vi "main(Test DQMH modules).bak.vi"() -> ()   [LabVIEW 2018, in "Application.lvlib"] (continued)
          tunnel: w8166 -> [w8203] mode=indexing
          tunnel: w8161 -> [w8204]
          tunnel: [w8200] -> w8164 mode=indexing
          n3766 = Unbundle By Name(w8203) -> ("command"=w8202:string, "command data"=w8201:variant)
          n3767 = call "App enquece.vi"("command data"=w8201, "command"=w8202, "queue in"=w8204) -> ("error out"=w8200:errorcluster)  [unwired: 7 in, 1 out]
        }
        n3768 = Merge Errors(w8165, w8164) -> (w8163:errorcluster)
      }
      frame "Test DRV 45A" {
        w8212 = T11 {"command"="", "command data"=variant} ("element")
        w8205 = 45 ("DUT index(0-59)")
        w8238 = T11 {"command"="", "command data"=variant} ("element")
        n3769 = disable-structure shown="LOGGING==TRUE" {
          disable-tunnel: w8216 -> [w8253 _]
          frame condition #0 (active) {
            n3770 = Empty String/Path?(string/path=w8253) -> (empty?=w8256:bool)
            n3771 = Select(t="Quece timeout", s=w8256, f=w8253) -> (s? t:f=w8252:string)
            n3772 = call "string log (SubVI).vi"("Enum"=enum16{"Init", "Log", "Read"}."Log", "state Name"=w8252) -> ()  [unwired: 8 in, 2 out]
          }
          frame condition #1 {
          }
        }
        n3773 = Flush Queue(queue=w8217) -> (queue out=w8218:refnum<queue>)  [unwired: 1 in, 2 out]
        n3774 = Decrement(x=w8205) -> (x-1=w8209:i32)
        n3775 = Index Array(array=w8206, index=w8209) -> (element=w8207:refnum<vi>)
        n3776 = property class="ColBox"(reference=w8207, "Value"=u32 10000536 ("DRV 1")) -> ()  [unwired: 1 in, 2 out]
        n3777 = To Variant(anything=bool[] [FALSE, FALSE, TRUE, FALSE, FALSE, FALSE]) -> (Variant=w8235:variant)
        n3778 = To Variant(anything=T6."demux1_10_channel8" ("demux1_10(x6)_encode")) -> (Variant=w8239:variant)
        n3779 = To Variant(anything=T4."mux6_1_channel3_3" ("mux6_1(3wires)_encode")) -> (Variant=w8242:variant)
        n3780 = To Variant(anything=T5."mux10_1_channel8" ("mux10_1(x6)_encode")) -> (Variant=w8244:variant)
        n3781 = Bundle By Name(cluster=w8238, "command"="MEAS.mux10-1", "command data"=w8244) -> (w8233:T11)
        n3782 = Bundle By Name(cluster=w8238, "command"="MEAS.mux6_1", "command data"=w8242) -> (w8232:T11)
        n3783 = Bundle By Name(cluster=w8238, "command"="MEAS.demux1-10", "command data"=w8239) -> (w8231:T11)
        n3784 = Bundle By Name(cluster=w8238, "command"="MEAS.eMIC", "command data"=w8235) -> (w8230:T11)
        n3785 = Bundle By Name(cluster=w8238, "command"="MEAS.AllRelaysOFF") -> (w8234:T11)
        n3786 = Build Array(w8234, w8233, w8232, w8231, w8230) -> (w8225:T11[])
        n3787 = Bundle By Name(cluster=w8212, "command"="MEAS.requestAC", "command data"=w8205) -> (w8226:T11)
        n3788 = Bundle By Name(cluster=w8212, "command"="Apps.WaitForEvent", "command data"=w8205) -> (w8211:T11)
        n3789 = Bundle By Name(cluster=w8212, "command"="MEAS.DMM dual read") -> (w8227:T11)
        n3790 = Bundle By Name(cluster=w8212, "command"="Apps.UI Update 1") -> (w8213:T11)
        n3791 = Build Array(w8227, w8226, w8211, w8213) -> (w8224:T11[])
        n3792 = Build Array (concatenate)(w8225, w8224) -> (w8223:T11[])
        n3793 = for {
          tunnel: w8223 -> [w8260] mode=indexing
          tunnel: w8218 -> [w8261]
          tunnel: [w8257] -> w8221 mode=indexing
          n3794 = Unbundle By Name(w8260) -> ("command"=w8259:string, "command data"=w8258:variant)
          n3795 = call "App enquece.vi"("command data"=w8258, "command"=w8259, "queue in"=w8261) -> ("error out"=w8257:errorcluster)  [unwired: 7 in, 1 out]
        }
        n3796 = Merge Errors(w8222, w8221) -> (w8220:errorcluster)
      }
      frame "Test DRV 46A" {
        w8269 = T11 {"command"="", "command data"=variant} ("element")
        w8263 = 46 ("DUT index(0-59)")
        w8295 = T11 {"command"="", "command data"=variant} ("element")
        n3797 = disable-structure shown="LOGGING==TRUE" {
          disable-tunnel: w8273 -> [w8310 _]
          frame condition #0 (active) {
            n3798 = Empty String/Path?(string/path=w8310) -> (empty?=w8313:bool)
            n3799 = Select(t="Quece timeout", s=w8313, f=w8310) -> (s? t:f=w8309:string)
            n3800 = call "string log (SubVI).vi"("Enum"=enum16{"Init", "Log", "Read"}."Log", "state Name"=w8309) -> ()  [unwired: 8 in, 2 out]
          }
          frame condition #1 {
          }
        }
        n3801 = Decrement(x=w8263) -> (x-1=w8266:i32)
        n3802 = Flush Queue(queue=w8274) -> (queue out=w8275:refnum<queue>)  [unwired: 1 in, 2 out]
        n3803 = Index Array(array=w8262, index=w8266) -> (element=w8264:refnum<vi>)
        n3804 = property class="ColBox"(reference=w8264, "Value"=u32 10000536 ("DRV 1")) -> ()  [unwired: 1 in, 2 out]
        n3805 = To Variant(anything=bool[] [FALSE, FALSE, TRUE, FALSE, FALSE, FALSE]) -> (Variant=w8292:variant)
        n3806 = To Variant(anything=T6."demux1_10_channel8" ("demux1_10(x6)_encode")) -> (Variant=w8296:variant)
        n3807 = To Variant(anything=T4."mux6_1_channel3_3" ("mux6_1(3wires)_encode")) -> (Variant=w8299:variant)
        n3808 = To Variant(anything=T5."mux10_1_channel8" ("mux10_1(x6)_encode")) -> (Variant=w8301:variant)
        n3809 = Bundle By Name(cluster=w8295, "command"="MEAS.mux10-1", "command data"=w8301) -> (w8290:T11)
        n3810 = Bundle By Name(cluster=w8295, "command"="MEAS.mux6_1", "command data"=w8299) -> (w8289:T11)
        n3811 = Bundle By Name(cluster=w8295, "command"="MEAS.demux1-10", "command data"=w8296) -> (w8288:T11)
        n3812 = Bundle By Name(cluster=w8295, "command"="MEAS.eMIC", "command data"=w8292) -> (w8287:T11)
        n3813 = Bundle By Name(cluster=w8295, "command"="MEAS.AllRelaysOFF") -> (w8291:T11)
        n3814 = Build Array(w8291, w8290, w8289, w8288, w8287) -> (w8282:T11[])
        n3815 = Bundle By Name(cluster=w8269, "command"="MEAS.requestAC", "command data"=w8263) -> (w8283:T11)
        n3816 = Bundle By Name(cluster=w8269, "command"="Apps.WaitForEvent", "command data"=w8263) -> (w8268:T11)
        n3817 = Bundle By Name(cluster=w8269, "command"="MEAS.DMM dual read") -> (w8284:T11)
        n3818 = Bundle By Name(cluster=w8269, "command"="Apps.UI Update 1") -> (w8270:T11)
        n3819 = Build Array(w8284, w8283, w8268, w8270) -> (w8281:T11[])
        n3820 = Build Array (concatenate)(w8282, w8281) -> (w8280:T11[])
        n3821 = for {
          tunnel: w8280 -> [w8317] mode=indexing
          tunnel: w8275 -> [w8318]
          tunnel: [w8314] -> w8278 mode=indexing
          n3822 = Unbundle By Name(w8317) -> ("command"=w8316:string, "command data"=w8315:variant)
          n3823 = call "App enquece.vi"("command data"=w8315, "command"=w8316, "queue in"=w8318) -> ("error out"=w8314:errorcluster)  [unwired: 7 in, 1 out]
        }
        n3824 = Merge Errors(w8279, w8278) -> (w8277:errorcluster)
      }
      frame "Test DRV 47A" {
        w8328 = T11 {"command"="", "command data"=variant} ("element")
        w8319 = 47 ("DUT index(0-59)")
        w8352 = T11 {"command"="", "command data"=variant} ("element")
        n3825 = disable-structure shown="LOGGING==TRUE" {
          disable-tunnel: w8332 -> [w8367 _]
          frame condition #0 (active) {
            n3826 = Empty String/Path?(string/path=w8367) -> (empty?=w8370:bool)
            n3827 = Select(t="Quece timeout", s=w8370, f=w8367) -> (s? t:f=w8366:string)
            n3828 = call "string log (SubVI).vi"("Enum"=enum16{"Init", "Log", "Read"}."Log", "state Name"=w8366) -> ()  [unwired: 8 in, 2 out]
          }
          frame condition #1 {
          }
        }
        n3829 = Decrement(x=w8319) -> (x-1=w8323:i32)
        n3830 = Flush Queue(queue=w8333) -> (queue out=w8334:refnum<queue>)  [unwired: 1 in, 2 out]
        n3831 = Index Array(array=w8320, index=w8323) -> (element=w8321:refnum<vi>)
        n3832 = property class="ColBox"(reference=w8321, "Value"=u32 10000536 ("DRV 1")) -> ()  [unwired: 1 in, 2 out]
        n3833 = To Variant(anything=bool[] [FALSE, FALSE, FALSE, FALSE, TRUE, FALSE]) -> (Variant=w8349:variant)
        n3834 = To Variant(anything=T6."demux1_10_channel8" ("demux1_10(x6)_encode")) -> (Variant=w8353:variant)
        n3835 = To Variant(anything=T4."mux6_1_channel5_3" ("mux6_1(3wires)_encode")) -> (Variant=w8356:variant)
        n3836 = To Variant(anything=T5."mux10_1_channel8" ("mux10_1(x6)_encode")) -> (Variant=w8358:variant)
        n3837 = Bundle By Name(cluster=w8352, "command"="MEAS.mux10-1", "command data"=w8358) -> (w8347:T11)
        n3838 = Bundle By Name(cluster=w8352, "command"="MEAS.mux6_1", "command data"=w8356) -> (w8346:T11)
        n3839 = Bundle By Name(cluster=w8352, "command"="MEAS.demux1-10", "command data"=w8353) -> (w8345:T11)
        n3840 = Bundle By Name(cluster=w8352, "command"="MEAS.eMIC", "command data"=w8349) -> (w8344:T11)
        n3841 = Bundle By Name(cluster=w8352, "command"="MEAS.AllRelaysOFF") -> (w8348:T11)
        n3842 = Build Array(w8348, w8347, w8346, w8345, w8344) -> (w8339:T11[])
        n3843 = Bundle By Name(cluster=w8328, "command"="MEAS.requestAC", "command data"=w8319) -> (w8340:T11)
        n3844 = Bundle By Name(cluster=w8328, "command"="Apps.WaitForEvent", "command data"=w8319) -> (w8327:T11)
        n3845 = Bundle By Name(cluster=w8328, "command"="Apps.UI Update 1") -> (w8329:T11)
        n3846 = Bundle By Name(cluster=w8328, "command"="MEAS.DMM dual read") -> (w8341:T11)
        n3847 = Build Array(w8341, w8340, w8327, w8329) -> (w8338:T11[])
        n3848 = Build Array (concatenate)(w8339, w8338) -> (w8337:T11[])
        n3849 = for {
          tunnel: w8337 -> [w8374] mode=indexing
          tunnel: w8334 -> [w8375]
          tunnel: [w8371] -> w8336 mode=indexing
          n3850 = Unbundle By Name(w8374) -> ("command"=w8373:string, "command data"=w8372:variant)
          n3851 = call "App enquece.vi"("command data"=w8372, "command"=w8373, "queue in"=w8375) -> ("error out"=w8371:errorcluster)  [unwired: 7 in, 1 out]
        }
        n3852 = Merge Errors(w8324, w8336) -> (w8335:errorcluster)
      }
      frame "Test DRV 48A" {
        w8383 = T11 {"command"="", "command data"=variant} ("element")
        w8377 = 48 ("DUT index(0-59)")
        w8409 = T11 {"command"="", "command data"=variant} ("element")
        n3853 = disable-structure shown="LOGGING==TRUE" {
          disable-tunnel: w8387 -> [w8424 _]
          frame condition #0 (active) {
            n3854 = Empty String/Path?(string/path=w8424) -> (empty?=w8427:bool)
            n3855 = Select(t="Quece timeout", s=w8427, f=w8424) -> (s? t:f=w8423:string)
            n3856 = call "string log (SubVI).vi"("Enum"=enum16{"Init", "Log", "Read"}."Log", "state Name"=w8423) -> ()  [unwired: 8 in, 2 out]
          }
          frame condition #1 {
          }
        }
        n3857 = Decrement(x=w8377) -> (x-1=w8380:i32)
        n3858 = Flush Queue(queue=w8388) -> (queue out=w8389:refnum<queue>)  [unwired: 1 in, 2 out]
        n3859 = Index Array(array=w8378, index=w8380) -> (element=w8376:refnum<vi>)
        n3860 = property class="ColBox"(reference=w8376, "Value"=u32 10000536 ("DRV 1")) -> ()  [unwired: 1 in, 2 out]
        n3861 = To Variant(anything=bool[] [FALSE, FALSE, FALSE, FALSE, FALSE, TRUE]) -> (Variant=w8406:variant)
        n3862 = To Variant(anything=T6."demux1_10_channel8" ("demux1_10(x6)_encode")) -> (Variant=w8410:variant)
        n3863 = To Variant(anything=T4."mux6_1_channel6_3" ("mux6_1(3wires)_encode")) -> (Variant=w8413:variant)
        n3864 = To Variant(anything=T5."mux10_1_channel8" ("mux10_1(x6)_encode")) -> (Variant=w8415:variant)
        n3865 = Bundle By Name(cluster=w8409, "command"="MEAS.mux10-1", "command data"=w8415) -> (w8404:T11)
        n3866 = Bundle By Name(cluster=w8409, "command"="MEAS.mux6_1", "command data"=w8413) -> (w8403:T11)
        n3867 = Bundle By Name(cluster=w8409, "command"="MEAS.demux1-10", "command data"=w8410) -> (w8402:T11)
        n3868 = Bundle By Name(cluster=w8409, "command"="MEAS.eMIC", "command data"=w8406) -> (w8401:T11)
        n3869 = Bundle By Name(cluster=w8409, "command"="MEAS.AllRelaysOFF") -> (w8405:T11)
        n3870 = Build Array(w8405, w8404, w8403, w8402, w8401) -> (w8396:T11[])
        n3871 = Bundle By Name(cluster=w8383, "command"="MEAS.requestAC", "command data"=w8377) -> (w8397:T11)
        n3872 = Bundle By Name(cluster=w8383, "command"="Apps.WaitForEvent", "command data"=w8377) -> (w8382:T11)
        n3873 = Bundle By Name(cluster=w8383, "command"="MEAS.DMM dual read") -> (w8398:T11)
        n3874 = Bundle By Name(cluster=w8383, "command"="Apps.UI Update 1") -> (w8384:T11)
        n3875 = Build Array(w8398, w8397, w8382, w8384) -> (w8395:T11[])
        n3876 = Build Array (concatenate)(w8396, w8395) -> (w8394:T11[])
        n3877 = for {
          tunnel: w8394 -> [w8431] mode=indexing
          tunnel: w8389 -> [w8432]
          tunnel: [w8428] -> w8392 mode=indexing
          n3878 = Unbundle By Name(w8431) -> ("command"=w8430:string, "command data"=w8429:variant)
          n3879 = call "App enquece.vi"("command data"=w8429, "command"=w8430, "queue in"=w8432) -> ("error out"=w8428:errorcluster)  [unwired: 7 in, 1 out]
        }
        n3880 = Merge Errors(w8393, w8392) -> (w8391:errorcluster)
      }
      frame "Test DRV 49A" {
        w8440 = T11 {"command"="", "command data"=variant} ("element")
        w8434 = 49 ("DUT index(0-59)")
        w8466 = T11 {"command"="", "command data"=variant} ("element")
        n3881 = disable-structure shown="LOGGING==TRUE" {
          disable-tunnel: w8444 -> [w8481 _]
          frame condition #0 (active) {
            n3882 = Empty String/Path?(string/path=w8481) -> (empty?=w8484:bool)
            n3883 = Select(t="Quece timeout", s=w8484, f=w8481) -> (s? t:f=w8480:string)
            n3884 = call "string log (SubVI).vi"("Enum"=enum16{"Init", "Log", "Read"}."Log", "state Name"=w8480) -> ()  [unwired: 8 in, 2 out]
          }
          frame condition #1 {
          }
        }
        n3885 = Flush Queue(queue=w8445) -> (queue out=w8446:refnum<queue>)  [unwired: 1 in, 2 out]
        n3886 = Decrement(x=w8434) -> (x-1=w8437:i32)
        n3887 = Index Array(array=w8435, index=w8437) -> (element=w8433:refnum<vi>)
        n3888 = property class="ColBox"(reference=w8433, "Value"=u32 10000536 ("DRV 1")) -> ()  [unwired: 1 in, 2 out]
        n3889 = To Variant(anything=bool[] [TRUE, FALSE, FALSE, FALSE, FALSE, FALSE]) -> (Variant=w8463:variant)
        n3890 = To Variant(anything=T6."demux1_10_channel9" ("demux1_10(x6)_encode")) -> (Variant=w8467:variant)
        n3891 = To Variant(anything=T4."mux6_1_channel1_3" ("mux6_1(3wires)_encode")) -> (Variant=w8470:variant)
        n3892 = To Variant(anything=T5."mux10_1_channel9" ("mux10_1(x6)_encode")) -> (Variant=w8472:variant)
        n3893 = Bundle By Name(cluster=w8466, "command"="MEAS.mux10-1", "command data"=w8472) -> (w8461:T11)
        n3894 = Bundle By Name(cluster=w8466, "command"="MEAS.mux6_1", "command data"=w8470) -> (w8460:T11)
        n3895 = Bundle By Name(cluster=w8466, "command"="MEAS.demux1-10", "command data"=w8467) -> (w8459:T11)
        n3896 = Bundle By Name(cluster=w8466, "command"="MEAS.eMIC", "command data"=w8463) -> (w8458:T11)
        n3897 = Bundle By Name(cluster=w8466, "command"="MEAS.AllRelaysOFF") -> (w8462:T11)
        n3898 = Build Array(w8462, w8461, w8460, w8459, w8458) -> (w8453:T11[])
        n3899 = Bundle By Name(cluster=w8440, "command"="MEAS.requestAC", "command data"=w8434) -> (w8454:T11)
        n3900 = Bundle By Name(cluster=w8440, "command"="Apps.WaitForEvent", "command data"=w8434) -> (w8439:T11)
        n3901 = Bundle By Name(cluster=w8440, "command"="MEAS.DMM dual read") -> (w8455:T11)
        n3902 = Bundle By Name(cluster=w8440, "command"="Apps.UI Update 1") -> (w8441:T11)
        n3903 = Build Array(w8455, w8454, w8439, w8441) -> (w8452:T11[])
        n3904 = Build Array (concatenate)(w8453, w8452) -> (w8451:T11[])
        n3905 = for {
          tunnel: w8451 -> [w8488] mode=indexing
          tunnel: w8446 -> [w8489]
          tunnel: [w8485] -> w8449 mode=indexing
          n3906 = Unbundle By Name(w8488) -> ("command"=w8487:string, "command data"=w8486:variant)
          n3907 = call "App enquece.vi"("command data"=w8486, "command"=w8487, "queue in"=w8489) -> ("error out"=w8485:errorcluster)  [unwired: 7 in, 1 out]
        }
        n3908 = Merge Errors(w8450, w8449) -> (w8448:errorcluster)
      }
      frame "Test DRV 50A" {
        w8497 = T11 {"command"="", "command data"=variant} ("element")
        w8491 = 50 ("DUT index(0-59)")
        w8523 = T11 {"command"="", "command data"=variant} ("element")
        n3909 = disable-structure shown="LOGGING==TRUE" {
          disable-tunnel: w8501 -> [w8538 _]
          frame condition #0 (active) {
            n3910 = Empty String/Path?(string/path=w8538) -> (empty?=w8541:bool)
            n3911 = Select(t="Quece timeout", s=w8541, f=w8538) -> (s? t:f=w8537:string)
            n3912 = call "string log (SubVI).vi"("Enum"=enum16{"Init", "Log", "Read"}."Log", "state Name"=w8537) -> ()  [unwired: 8 in, 2 out]
          }
          frame condition #1 {
          }
        }
        n3913 = Flush Queue(queue=w8502) -> (queue out=w8503:refnum<queue>)  [unwired: 1 in, 2 out]
        n3914 = Decrement(x=w8491) -> (x-1=w8494:i32)
        n3915 = Index Array(array=w8492, index=w8494) -> (element=w8490:refnum<vi>)
        n3916 = property class="ColBox"(reference=w8490, "Value"=u32 10000536 ("DRV 1")) -> ()  [unwired: 1 in, 2 out]
        n3917 = To Variant(anything=bool[] [FALSE, TRUE, FALSE, FALSE, FALSE, FALSE]) -> (Variant=w8520:variant)
        n3918 = To Variant(anything=T6."demux1_10_channel9" ("demux1_10(x6)_encode")) -> (Variant=w8524:variant)
        n3919 = To Variant(anything=T4."mux6_1_channel2_3" ("mux6_1(3wires)_encode")) -> (Variant=w8527:variant)
        n3920 = To Variant(anything=T5."mux10_1_channel9" ("mux10_1(x6)_encode")) -> (Variant=w8529:variant)
        n3921 = Bundle By Name(cluster=w8523, "command"="MEAS.mux10-1", "command data"=w8529) -> (w8518:T11)
        n3922 = Bundle By Name(cluster=w8523, "command"="MEAS.mux6_1", "command data"=w8527) -> (w8517:T11)
        n3923 = Bundle By Name(cluster=w8523, "command"="MEAS.demux1-10", "command data"=w8524) -> (w8516:T11)
        n3924 = Bundle By Name(cluster=w8523, "command"="MEAS.eMIC", "command data"=w8520) -> (w8515:T11)
        n3925 = Bundle By Name(cluster=w8523, "command"="MEAS.AllRelaysOFF") -> (w8519:T11)
        n3926 = Build Array(w8519, w8518, w8517, w8516, w8515) -> (w8510:T11[])
        n3927 = Bundle By Name(cluster=w8497, "command"="MEAS.requestAC", "command data"=w8491) -> (w8511:T11)
        n3928 = Bundle By Name(cluster=w8497, "command"="Apps.WaitForEvent", "command data"=w8491) -> (w8496:T11)
        n3929 = Bundle By Name(cluster=w8497, "command"="MEAS.DMM dual read") -> (w8512:T11)
        n3930 = Bundle By Name(cluster=w8497, "command"="Apps.UI Update 1") -> (w8498:T11)
        n3931 = Build Array(w8512, w8511, w8496, w8498) -> (w8509:T11[])
        n3932 = Build Array (concatenate)(w8510, w8509) -> (w8508:T11[])
        n3933 = for {
          tunnel: w8508 -> [w8545] mode=indexing
          tunnel: w8503 -> [w8546]
          tunnel: [w8542] -> w8506 mode=indexing
          n3934 = Unbundle By Name(w8545) -> ("command"=w8544:string, "command data"=w8543:variant)
          n3935 = call "App enquece.vi"("command data"=w8543, "command"=w8544, "queue in"=w8546) -> ("error out"=w8542:errorcluster)  [unwired: 7 in, 1 out]
        }
        n3936 = Merge Errors(w8507, w8506) -> (w8505:errorcluster)
      }
      frame "Test DRV 51A" {
        w8554 = T11 {"command"="", "command data"=variant} ("element")
        w8547 = 51 ("DUT index(0-59)")
        w8580 = T11 {"command"="", "command data"=variant} ("element")
        n3937 = disable-structure shown="LOGGING==TRUE" {
          disable-tunnel: w8558 -> [w8595 _]
          frame condition #0 (active) {
            n3938 = Empty String/Path?(string/path=w8595) -> (empty?=w8598:bool)
            n3939 = Select(t="Quece timeout", s=w8598, f=w8595) -> (s? t:f=w8594:string)
            n3940 = call "string log (SubVI).vi"("Enum"=enum16{"Init", "Log", "Read"}."Log", "state Name"=w8594) -> ()  [unwired: 8 in, 2 out]
          }
          frame condition #1 {
          }
        }
        n3941 = Flush Queue(queue=w8559) -> (queue out=w8560:refnum<queue>)  [unwired: 1 in, 2 out]
        n3942 = Decrement(x=w8547) -> (x-1=w8551:i32)
        n3943 = Index Array(array=w8548, index=w8551) -> (element=w8549:refnum<vi>)
        n3944 = property class="ColBox"(reference=w8549, "Value"=u32 10000536 ("DRV 1")) -> ()  [unwired: 1 in, 2 out]
        n3945 = To Variant(anything=bool[] [FALSE, FALSE, TRUE, FALSE, FALSE, FALSE]) -> (Variant=w8577:variant)
        n3946 = To Variant(anything=T6."demux1_10_channel9" ("demux1_10(x6)_encode")) -> (Variant=w8581:variant)
        n3947 = To Variant(anything=T4."mux6_1_channel3_3" ("mux6_1(3wires)_encode")) -> (Variant=w8584:variant)
        n3948 = To Variant(anything=T5."mux10_1_channel9" ("mux10_1(x6)_encode")) -> (Variant=w8586:variant)
        n3949 = Bundle By Name(cluster=w8580, "command"="MEAS.mux10-1", "command data"=w8586) -> (w8575:T11)
        n3950 = Bundle By Name(cluster=w8580, "command"="MEAS.mux6_1", "command data"=w8584) -> (w8574:T11)
        n3951 = Bundle By Name(cluster=w8580, "command"="MEAS.demux1-10", "command data"=w8581) -> (w8573:T11)
        n3952 = Bundle By Name(cluster=w8580, "command"="MEAS.eMIC", "command data"=w8577) -> (w8572:T11)
        n3953 = Bundle By Name(cluster=w8580, "command"="MEAS.AllRelaysOFF") -> (w8576:T11)
        n3954 = Build Array(w8576, w8575, w8574, w8573, w8572) -> (w8567:T11[])
        n3955 = Bundle By Name(cluster=w8554, "command"="MEAS.requestAC", "command data"=w8547) -> (w8568:T11)
        n3956 = Bundle By Name(cluster=w8554, "command"="Apps.WaitForEvent", "command data"=w8547) -> (w8553:T11)
        n3957 = Bundle By Name(cluster=w8554, "command"="MEAS.DMM dual read") -> (w8569:T11)
        n3958 = Bundle By Name(cluster=w8554, "command"="Apps.UI Update 1") -> (w8555:T11)
        n3959 = Build Array(w8569, w8568, w8553, w8555) -> (w8566:T11[])
        n3960 = Build Array (concatenate)(w8567, w8566) -> (w8565:T11[])
        n3961 = for {
          tunnel: w8565 -> [w8602] mode=indexing
          tunnel: w8560 -> [w8603]
          tunnel: [w8599] -> w8563 mode=indexing
          n3962 = Unbundle By Name(w8602) -> ("command"=w8601:string, "command data"=w8600:variant)
          n3963 = call "App enquece.vi"("command data"=w8600, "command"=w8601, "queue in"=w8603) -> ("error out"=w8599:errorcluster)  [unwired: 7 in, 1 out]
        }
        n3964 = Merge Errors(w8564, w8563) -> (w8562:errorcluster)
      }
      frame "Test DRV 52A" {
        w8611 = T11 {"command"="", "command data"=variant} ("element")
        w8604 = 52 ("DUT index(0-59)")
        w8637 = T11 {"command"="", "command data"=variant} ("element")
        n3965 = disable-structure shown="LOGGING==TRUE" {
          disable-tunnel: w8615 -> [w8652 _]
          frame condition #0 (active) {
            n3966 = Empty String/Path?(string/path=w8652) -> (empty?=w8655:bool)
            n3967 = Select(t="Quece timeout", s=w8655, f=w8652) -> (s? t:f=w8651:string)
            n3968 = call "string log (SubVI).vi"("Enum"=enum16{"Init", "Log", "Read"}."Log", "state Name"=w8651) -> ()  [unwired: 8 in, 2 out]
          }
          frame condition #1 {
          }
        }
        n3969 = Flush Queue(queue=w8616) -> (queue out=w8617:refnum<queue>)  [unwired: 1 in, 2 out]
        n3970 = Decrement(x=w8604) -> (x-1=w8608:i32)
        n3971 = Index Array(array=w8605, index=w8608) -> (element=w8606:refnum<vi>)
        n3972 = property class="ColBox"(reference=w8606, "Value"=u32 10000536 ("DRV 1")) -> ()  [unwired: 1 in, 2 out]
        n3973 = To Variant(anything=bool[] [FALSE, FALSE, FALSE, TRUE, FALSE, FALSE]) -> (Variant=w8634:variant)
        n3974 = To Variant(anything=T6."demux1_10_channel9" ("demux1_10(x6)_encode")) -> (Variant=w8638:variant)
        n3975 = To Variant(anything=T4."mux6_1_channel4_3" ("mux6_1(3wires)_encode")) -> (Variant=w8641:variant)
        n3976 = To Variant(anything=T5."mux10_1_channel9" ("mux10_1(x6)_encode")) -> (Variant=w8643:variant)
        n3977 = Bundle By Name(cluster=w8637, "command"="MEAS.mux10-1", "command data"=w8643) -> (w8632:T11)
        n3978 = Bundle By Name(cluster=w8637, "command"="MEAS.mux6_1", "command data"=w8641) -> (w8631:T11)
        n3979 = Bundle By Name(cluster=w8637, "command"="MEAS.demux1-10", "command data"=w8638) -> (w8630:T11)
        n3980 = Bundle By Name(cluster=w8637, "command"="MEAS.eMIC", "command data"=w8634) -> (w8629:T11)
        n3981 = Bundle By Name(cluster=w8637, "command"="MEAS.AllRelaysOFF") -> (w8633:T11)
        n3982 = Build Array(w8633, w8632, w8631, w8630, w8629) -> (w8624:T11[])
        n3983 = Bundle By Name(cluster=w8611, "command"="MEAS.requestAC", "command data"=w8604) -> (w8625:T11)
        n3984 = Bundle By Name(cluster=w8611, "command"="Apps.WaitForEvent", "command data"=w8604) -> (w8610:T11)
        n3985 = Bundle By Name(cluster=w8611, "command"="MEAS.DMM dual read") -> (w8626:T11)
        n3986 = Bundle By Name(cluster=w8611, "command"="Apps.UI Update 1") -> (w8612:T11)
        n3987 = Build Array(w8626, w8625, w8610, w8612) -> (w8623:T11[])
        n3988 = Build Array (concatenate)(w8624, w8623) -> (w8622:T11[])
        n3989 = for {
          tunnel: w8622 -> [w8659] mode=indexing
          tunnel: w8617 -> [w8660]
          tunnel: [w8656] -> w8620 mode=indexing
          n3990 = Unbundle By Name(w8659) -> ("command"=w8658:string, "command data"=w8657:variant)
          n3991 = call "App enquece.vi"("command data"=w8657, "command"=w8658, "queue in"=w8660) -> ("error out"=w8656:errorcluster)  [unwired: 7 in, 1 out]
        }
        n3992 = Merge Errors(w8621, w8620) -> (w8619:errorcluster)
      }
      frame "Test DRV 53A" {
        w8669 = T11 {"command"="", "command data"=variant} ("element")
        w8661 = 53 ("DUT index(0-59)")
        w8694 = T11 {"command"="", "command data"=variant} ("element")
        n3993 = disable-structure shown="LOGGING==TRUE" {
          disable-tunnel: w8673 -> [w8709 _]
          frame condition #0 (active) {
            n3994 = Empty String/Path?(string/path=w8709) -> (empty?=w8712:bool)
            n3995 = Select(t="Quece timeout", s=w8712, f=w8709) -> (s? t:f=w8708:string)
            n3996 = call "string log (SubVI).vi"("Enum"=enum16{"Init", "Log", "Read"}."Log", "state Name"=w8708) -> ()  [unwired: 8 in, 2 out]
          }
          frame condition #1 {
          }
        }
        n3997 = Flush Queue(queue=w8674) -> (queue out=w8675:refnum<queue>)  [unwired: 1 in, 2 out]
        n3998 = Decrement(x=w8661) -> (x-1=w8665:i32)
        n3999 = Index Array(array=w8662, index=w8665) -> (element=w8663:refnum<vi>)
        n4000 = property class="ColBox"(reference=w8663, "Value"=u32 10000536 ("DRV 1")) -> ()  [unwired: 1 in, 2 out]
        n4001 = To Variant(anything=bool[] [FALSE, FALSE, FALSE, FALSE, TRUE, FALSE]) -> (Variant=w8691:variant)
        n4002 = To Variant(anything=T6."demux1_10_channel9" ("demux1_10(x6)_encode")) -> (Variant=w8695:variant)
        n4003 = To Variant(anything=T4."mux6_1_channel5_3" ("mux6_1(3wires)_encode")) -> (Variant=w8698:variant)
        n4004 = To Variant(anything=T5."mux10_1_channel9" ("mux10_1(x6)_encode")) -> (Variant=w8700:variant)
        n4005 = Bundle By Name(cluster=w8694, "command"="MEAS.mux10-1", "command data"=w8700) -> (w8689:T11)
        n4006 = Bundle By Name(cluster=w8694, "command"="MEAS.mux6_1", "command data"=w8698) -> (w8688:T11)
        n4007 = Bundle By Name(cluster=w8694, "command"="MEAS.demux1-10", "command data"=w8695) -> (w8687:T11)
        n4008 = Bundle By Name(cluster=w8694, "command"="MEAS.eMIC", "command data"=w8691) -> (w8686:T11)
        n4009 = Bundle By Name(cluster=w8694, "command"="MEAS.AllRelaysOFF") -> (w8690:T11)
        n4010 = Build Array(w8690, w8689, w8688, w8687, w8686) -> (w8682:T11[])
        n4011 = Bundle By Name(cluster=w8669, "command"="MEAS.requestAC", "command data"=w8661) -> (w8683:T11)
        n4012 = Bundle By Name(cluster=w8669, "command"="Apps.WaitForEvent", "command data"=w8661) -> (w8668:T11)
        n4013 = Bundle By Name(cluster=w8669, "command"="MEAS.DMM dual read") -> (w8684:T11)
        n4014 = Bundle By Name(cluster=w8669, "command"="Apps.UI Update 1") -> (w8670:T11)
        n4015 = Build Array(w8684, w8683, w8668, w8670) -> (w8681:T11[])
        n4016 = Build Array (concatenate)(w8682, w8681) -> (w8680:T11[])
        n4017 = for {
          tunnel: w8680 -> [w8716] mode=indexing
          tunnel: w8675 -> [w8717]
          tunnel: [w8713] -> w8678 mode=indexing
          n4018 = Unbundle By Name(w8716) -> ("command"=w8715:string, "command data"=w8714:variant)
          n4019 = call "App enquece.vi"("command data"=w8714, "command"=w8715, "queue in"=w8717) -> ("error out"=w8713:errorcluster)  [unwired: 7 in, 1 out]
        }
        n4020 = Merge Errors(w8679, w8678) -> (w8677:errorcluster)
      }
      frame "Test DRV 54A" {
        w8725 = T11 {"command"="", "command data"=variant} ("element")
        w8718 = 54 ("DUT index(0-59)")
        w8751 = T11 {"command"="", "command data"=variant} ("element")
        n4021 = disable-structure shown="LOGGING==TRUE" {
          disable-tunnel: w8729 -> [w8766 _]
          frame condition #0 (active) {
            n4022 = Empty String/Path?(string/path=w8766) -> (empty?=w8769:bool)
            n4023 = Select(t="Quece timeout", s=w8769, f=w8766) -> (s? t:f=w8765:string)
            n4024 = call "string log (SubVI).vi"("Enum"=enum16{"Init", "Log", "Read"}."Log", "state Name"=w8765) -> ()  [unwired: 8 in, 2 out]
          }
          frame condition #1 {
          }
        }
        n4025 = Flush Queue(queue=w8730) -> (queue out=w8731:refnum<queue>)  [unwired: 1 in, 2 out]
        n4026 = Decrement(x=w8718) -> (x-1=w8722:i32)
        n4027 = Index Array(array=w8719, index=w8722) -> (element=w8720:refnum<vi>)
        n4028 = property class="ColBox"(reference=w8720, "Value"=u32 10000536 ("DRV 1")) -> ()  [unwired: 1 in, 2 out]
        n4029 = To Variant(anything=bool[] [FALSE, FALSE, FALSE, FALSE, FALSE, TRUE]) -> (Variant=w8748:variant)
        n4030 = To Variant(anything=T6."demux1_10_channel9" ("demux1_10(x6)_encode")) -> (Variant=w8752:variant)
        n4031 = To Variant(anything=T4."mux6_1_channel6_3" ("mux6_1(3wires)_encode")) -> (Variant=w8755:variant)
        n4032 = To Variant(anything=T5."mux10_1_channel9" ("mux10_1(x6)_encode")) -> (Variant=w8757:variant)
        n4033 = Bundle By Name(cluster=w8751, "command"="MEAS.mux10-1", "command data"=w8757) -> (w8746:T11)
        n4034 = Bundle By Name(cluster=w8751, "command"="MEAS.mux6_1", "command data"=w8755) -> (w8745:T11)
        n4035 = Bundle By Name(cluster=w8751, "command"="MEAS.demux1-10", "command data"=w8752) -> (w8744:T11)
        n4036 = Bundle By Name(cluster=w8751, "command"="MEAS.eMIC", "command data"=w8748) -> (w8743:T11)
        n4037 = Bundle By Name(cluster=w8751, "command"="MEAS.AllRelaysOFF") -> (w8747:T11)
        n4038 = Build Array(w8747, w8746, w8745, w8744, w8743) -> (w8738:T11[])
        n4039 = Bundle By Name(cluster=w8725, "command"="MEAS.requestAC", "command data"=w8718) -> (w8739:T11)
        n4040 = Bundle By Name(cluster=w8725, "command"="Apps.WaitForEvent", "command data"=w8718) -> (w8724:T11)
        n4041 = Bundle By Name(cluster=w8725, "command"="MEAS.DMM dual read") -> (w8740:T11)
        n4042 = Bundle By Name(cluster=w8725, "command"="Apps.UI Update 1") -> (w8726:T11)
        n4043 = Build Array(w8740, w8739, w8724, w8726) -> (w8737:T11[])
        n4044 = Build Array (concatenate)(w8738, w8737) -> (w8736:T11[])
        n4045 = for {
          tunnel: w8736 -> [w8773] mode=indexing
          tunnel: w8731 -> [w8774]
          tunnel: [w8770] -> w8734 mode=indexing
          n4046 = Unbundle By Name(w8773) -> ("command"=w8772:string, "command data"=w8771:variant)
          n4047 = call "App enquece.vi"("command data"=w8771, "command"=w8772, "queue in"=w8774) -> ("error out"=w8770:errorcluster)  [unwired: 7 in, 1 out]
        }
        n4048 = Merge Errors(w8735, w8734) -> (w8733:errorcluster)
      }
      frame "Test DRV 55A" {
        w8782 = T11 {"command"="", "command data"=variant} ("element")
        w8775 = 55 ("DUT index(0-59)")
        w8808 = T11 {"command"="", "command data"=variant} ("element")
        n4049 = disable-structure shown="LOGGING==TRUE" {
          disable-tunnel: w8786 -> [w8823 _]
          frame condition #0 (active) {
            n4050 = Empty String/Path?(string/path=w8823) -> (empty?=w8826:bool)
            n4051 = Select(t="Quece timeout", s=w8826, f=w8823) -> (s? t:f=w8822:string)
            n4052 = call "string log (SubVI).vi"("Enum"=enum16{"Init", "Log", "Read"}."Log", "state Name"=w8822) -> ()  [unwired: 8 in, 2 out]
          }
          frame condition #1 {
          }
        }
        n4053 = Flush Queue(queue=w8787) -> (queue out=w8788:refnum<queue>)  [unwired: 1 in, 2 out]
        n4054 = Decrement(x=w8775) -> (x-1=w8779:i32)
        n4055 = Index Array(array=w8776, index=w8779) -> (element=w8777:refnum<vi>)
        n4056 = property class="ColBox"(reference=w8777, "Value"=u32 10000536 ("DRV 1")) -> ()  [unwired: 1 in, 2 out]
        n4057 = To Variant(anything=bool[] [TRUE, FALSE, FALSE, FALSE, FALSE, FALSE]) -> (Variant=w8805:variant)
        n4058 = To Variant(anything=T6."demux1_10_channel10" ("demux1_10(x6)_encode")) -> (Variant=w8809:variant)
        n4059 = To Variant(anything=T4."mux6_1_channel1_3" ("mux6_1(3wires)_encode")) -> (Variant=w8812:variant)
        n4060 = To Variant(anything=T5."mux10_1_channel10" ("mux10_1(x6)_encode")) -> (Variant=w8814:variant)
        n4061 = Bundle By Name(cluster=w8808, "command"="MEAS.mux10-1", "command data"=w8814) -> (w8803:T11)
        n4062 = Bundle By Name(cluster=w8808, "command"="MEAS.mux6_1", "command data"=w8812) -> (w8802:T11)
        n4063 = Bundle By Name(cluster=w8808, "command"="MEAS.demux1-10", "command data"=w8809) -> (w8801:T11)
        n4064 = Bundle By Name(cluster=w8808, "command"="MEAS.eMIC", "command data"=w8805) -> (w8800:T11)
        n4065 = Bundle By Name(cluster=w8808, "command"="MEAS.AllRelaysOFF") -> (w8804:T11)
        n4066 = Build Array(w8804, w8803, w8802, w8801, w8800) -> (w8795:T11[])
        n4067 = Bundle By Name(cluster=w8782, "command"="MEAS.requestAC", "command data"=w8775) -> (w8796:T11)
        n4068 = Bundle By Name(cluster=w8782, "command"="Apps.WaitForEvent", "command data"=w8775) -> (w8781:T11)
        n4069 = Bundle By Name(cluster=w8782, "command"="MEAS.DMM dual read") -> (w8797:T11)
        n4070 = Bundle By Name(cluster=w8782, "command"="Apps.UI Update 1") -> (w8783:T11)
        n4071 = Build Array(w8797, w8796, w8781, w8783) -> (w8794:T11[])
        n4072 = Build Array (concatenate)(w8795, w8794) -> (w8793:T11[])
        n4073 = for {
          tunnel: w8793 -> [w8830] mode=indexing
          tunnel: w8788 -> [w8831]
          tunnel: [w8827] -> w8791 mode=indexing
          n4074 = Unbundle By Name(w8830) -> ("command"=w8829:string, "command data"=w8828:variant)
          n4075 = call "App enquece.vi"("command data"=w8828, "command"=w8829, "queue in"=w8831) -> ("error out"=w8827:errorcluster)  [unwired: 7 in, 1 out]
        }
        n4076 = Merge Errors(w8792, w8791) -> (w8790:errorcluster)
      }
      frame "Test DRV 56A" {
        w8839 = T11 {"command"="", "command data"=variant} ("element")
        w8832 = 56 ("DUT index(0-59)")
        w8865 = T11 {"command"="", "command data"=variant} ("element")
        n4077 = disable-structure shown="LOGGING==TRUE" {
          disable-tunnel: w8843 -> [w8880 _]
          frame condition #0 (active) {
            n4078 = Empty String/Path?(string/path=w8880) -> (empty?=w8883:bool)
            n4079 = Select(t="Quece timeout", s=w8883, f=w8880) -> (s? t:f=w8879:string)
            n4080 = call "string log (SubVI).vi"("Enum"=enum16{"Init", "Log", "Read"}."Log", "state Name"=w8879) -> ()  [unwired: 8 in, 2 out]
          }
          frame condition #1 {
          }
        }
        n4081 = Flush Queue(queue=w8844) -> (queue out=w8845:refnum<queue>)  [unwired: 1 in, 2 out]
        n4082 = Decrement(x=w8832) -> (x-1=w8836:i32)
        n4083 = Index Array(array=w8833, index=w8836) -> (element=w8834:refnum<vi>)
        n4084 = property class="ColBox"(reference=w8834, "Value"=u32 10000536 ("DRV 1")) -> ()  [unwired: 1 in, 2 out]
        n4085 = To Variant(anything=bool[] [FALSE, TRUE, FALSE, FALSE, FALSE, FALSE]) -> (Variant=w8862:variant)
        n4086 = To Variant(anything=T6."demux1_10_channel10" ("demux1_10(x6)_encode")) -> (Variant=w8866:variant)
        n4087 = To Variant(anything=T4."mux6_1_channel2_3" ("mux6_1(3wires)_encode")) -> (Variant=w8869:variant)
        n4088 = To Variant(anything=T5."mux10_1_channel10" ("mux10_1(x6)_encode")) -> (Variant=w8871:variant)
        n4089 = Bundle By Name(cluster=w8865, "command"="MEAS.mux10-1", "command data"=w8871) -> (w8860:T11)
        n4090 = Bundle By Name(cluster=w8865, "command"="MEAS.mux6_1", "command data"=w8869) -> (w8859:T11)
        n4091 = Bundle By Name(cluster=w8865, "command"="MEAS.demux1-10", "command data"=w8866) -> (w8858:T11)
        n4092 = Bundle By Name(cluster=w8865, "command"="MEAS.eMIC", "command data"=w8862) -> (w8857:T11)
        n4093 = Bundle By Name(cluster=w8865, "command"="MEAS.AllRelaysOFF") -> (w8861:T11)
        n4094 = Build Array(w8861, w8860, w8859, w8858, w8857) -> (w8852:T11[])
        n4095 = Bundle By Name(cluster=w8839, "command"="MEAS.requestAC", "command data"=w8832) -> (w8853:T11)
        n4096 = Bundle By Name(cluster=w8839, "command"="Apps.WaitForEvent", "command data"=w8832) -> (w8838:T11)
        n4097 = Bundle By Name(cluster=w8839, "command"="MEAS.DMM dual read") -> (w8854:T11)
        n4098 = Bundle By Name(cluster=w8839, "command"="Apps.UI Update 1") -> (w8840:T11)
        n4099 = Build Array(w8854, w8853, w8838, w8840) -> (w8851:T11[])
        n4100 = Build Array (concatenate)(w8852, w8851) -> (w8850:T11[])
        n4101 = for {
          tunnel: w8850 -> [w8887] mode=indexing
          tunnel: w8845 -> [w8888]
          tunnel: [w8884] -> w8848 mode=indexing
          n4102 = Unbundle By Name(w8887) -> ("command"=w8886:string, "command data"=w8885:variant)
          n4103 = call "App enquece.vi"("command data"=w8885, "command"=w8886, "queue in"=w8888) -> ("error out"=w8884:errorcluster)  [unwired: 7 in, 1 out]
        }
        n4104 = Merge Errors(w8849, w8848) -> (w8847:errorcluster)
      }
      frame "Test DRV 57A" {
        w8892 = T11 {"command"="", "command data"=variant} ("element")
        w8893 = 57 ("DUT index(0-59)")
        w8924 = T11 {"command"="", "command data"=variant} ("element")
        n4105 = disable-structure shown="LOGGING==TRUE" {
          disable-tunnel: w8903 -> [w8939 _]
          frame condition #0 (active) {
            n4106 = Empty String/Path?(string/path=w8939) -> (empty?=w8942:bool)
            n4107 = Select(t="Quece timeout", s=w8942, f=w8939) -> (s? t:f=w8938:string)
            n4108 = call "string log (SubVI).vi"("Enum"=enum16{"Init", "Log", "Read"}."Log", "state Name"=w8938) -> ()  [unwired: 8 in, 2 out]
          }
          frame condition #1 {
          }
        }
        n4109 = Flush Queue(queue=w8904) -> (queue out=w8905:refnum<queue>)  [unwired: 1 in, 2 out]
        n4110 = Decrement(x=w8893) -> (x-1=w8897:i32)
        n4111 = Index Array(array=w8894, index=w8897) -> (element=w8895:refnum<vi>)
        n4112 = property class="ColBox"(reference=w8895, "Value"=u32 10000536 ("DRV 1")) -> ()  [unwired: 1 in, 2 out]
        n4113 = To Variant(anything=bool[] [FALSE, FALSE, TRUE, FALSE, FALSE, FALSE]) -> (Variant=w8921:variant)
        n4114 = To Variant(anything=T6."demux1_10_channel10" ("demux1_10(x6)_encode")) -> (Variant=w8925:variant)
        n4115 = To Variant(anything=T4."mux6_1_channel3_3" ("mux6_1(3wires)_encode")) -> (Variant=w8928:variant)
        n4116 = To Variant(anything=T5."mux10_1_channel10" ("mux10_1(x6)_encode")) -> (Variant=w8930:variant)
        n4117 = Bundle By Name(cluster=w8924, "command"="MEAS.mux10-1", "command data"=w8930) -> (w8919:T11)
        n4118 = Bundle By Name(cluster=w8924, "command"="MEAS.mux6_1", "command data"=w8928) -> (w8918:T11)
        n4119 = Bundle By Name(cluster=w8924, "command"="MEAS.demux1-10", "command data"=w8925) -> (w8917:T11)
        n4120 = Bundle By Name(cluster=w8924, "command"="MEAS.eMIC", "command data"=w8921) -> (w8916:T11)
        n4121 = Bundle By Name(cluster=w8924, "command"="MEAS.AllRelaysOFF") -> (w8920:T11)
        n4122 = Build Array(w8920, w8919, w8918, w8917, w8916) -> (w8912:T11[])
        n4123 = Bundle By Name(cluster=w8892, "command"="MEAS.requestAC", "command data"=w8893) -> (w8913:T11)
        n4124 = Bundle By Name(cluster=w8892, "command"="Apps.WaitForEvent", "command data"=w8893) -> (w8899:T11)
        n4125 = Bundle By Name(cluster=w8892, "command"="MEAS.DMM dual read") -> (w8890:T11)
        n4126 = Bundle By Name(cluster=w8892, "command"="WaitFor") -> (w8889:T11)
        n4127 = Bundle By Name(cluster=w8892, "command"="Apps.UI Update 1") -> (w8900:T11)
        n4128 = Build Array(w8890, w8889, w8913, w8899, w8900) -> (w8911:T11[])
        n4129 = Build Array (concatenate)(w8912, w8911) -> (w8910:T11[])
        n4130 = for {
          tunnel: w8910 -> [w8946] mode=indexing
          tunnel: w8905 -> [w8947]
          tunnel: [w8943] -> w8908 mode=indexing
          n4131 = Unbundle By Name(w8946) -> ("command"=w8945:string, "command data"=w8944:variant)
          n4132 = call "App enquece.vi"("command data"=w8944, "command"=w8945, "queue in"=w8947) -> ("error out"=w8943:errorcluster)  [unwired: 7 in, 1 out]
        }
        n4133 = Merge Errors(w8909, w8908) -> (w8907:errorcluster)
      }
      frame "Test DRV 58A" {
        w8951 = T11 {"command"="", "command data"=variant} ("element")
        w8952 = 58 ("DUT index(0-59)")
        w8983 = T11 {"command"="", "command data"=variant} ("element")
        n4134 = disable-structure shown="LOGGING==TRUE" {
          disable-tunnel: w8962 -> [w8998 _]
          frame condition #0 (active) {
            n4135 = Empty String/Path?(string/path=w8998) -> (empty?=w9001:bool)
            n4136 = Select(t="Quece timeout", s=w9001, f=w8998) -> (s? t:f=w8997:string)
            n4137 = call "string log (SubVI).vi"("Enum"=enum16{"Init", "Log", "Read"}."Log", "state Name"=w8997) -> ()  [unwired: 8 in, 2 out]
          }
          frame condition #1 {
          }
        }
        n4138 = Flush Queue(queue=w8963) -> (queue out=w8964:refnum<queue>)  [unwired: 1 in, 2 out]
        n4139 = Decrement(x=w8952) -> (x-1=w8956:i32)
        n4140 = Index Array(array=w8953, index=w8956) -> (element=w8954:refnum<vi>)
        n4141 = property class="ColBox"(reference=w8954, "Value"=u32 10000536 ("DRV 1")) -> ()  [unwired: 1 in, 2 out]
        n4142 = To Variant(anything=bool[] [FALSE, FALSE, FALSE, TRUE, FALSE, FALSE]) -> (Variant=w8980:variant)
        n4143 = To Variant(anything=T6."demux1_10_channel10" ("demux1_10(x6)_encode")) -> (Variant=w8984:variant)
        n4144 = To Variant(anything=T4."mux6_1_channel4_3" ("mux6_1(3wires)_encode")) -> (Variant=w8987:variant)
        n4145 = To Variant(anything=T5."mux10_1_channel10" ("mux10_1(x6)_encode")) -> (Variant=w8989:variant)
        n4146 = Bundle By Name(cluster=w8983, "command"="MEAS.mux10-1", "command data"=w8989) -> (w8978:T11)
        n4147 = Bundle By Name(cluster=w8983, "command"="MEAS.mux6_1", "command data"=w8987) -> (w8977:T11)
        n4148 = Bundle By Name(cluster=w8983, "command"="MEAS.demux1-10", "command data"=w8984) -> (w8976:T11)
        n4149 = Bundle By Name(cluster=w8983, "command"="MEAS.eMIC", "command data"=w8980) -> (w8975:T11)
        n4150 = Bundle By Name(cluster=w8983, "command"="MEAS.AllRelaysOFF") -> (w8979:T11)
        n4151 = Build Array(w8979, w8978, w8977, w8976, w8975) -> (w8971:T11[])
        n4152 = Bundle By Name(cluster=w8951, "command"="MEAS.requestAC", "command data"=w8952) -> (w8972:T11)
        n4153 = Bundle By Name(cluster=w8951, "command"="Apps.WaitForEvent", "command data"=w8952) -> (w8958:T11)
        n4154 = Bundle By Name(cluster=w8951, "command"="MEAS.DMM dual read") -> (w8950:T11)
        n4155 = Bundle By Name(cluster=w8951, "command"="WaitFor") -> (w8949:T11)
        n4156 = Bundle By Name(cluster=w8951, "command"="Apps.UI Update 1") -> (w8959:T11)
        n4157 = Build Array(w8950, w8949, w8972, w8958, w8959) -> (w8970:T11[])
        n4158 = Build Array (concatenate)(w8971, w8970) -> (w8969:T11[])
        n4159 = for {
          tunnel: w8969 -> [w9005] mode=indexing
          tunnel: w8964 -> [w9006]
          tunnel: [w9002] -> w8967 mode=indexing
          n4160 = Unbundle By Name(w9005) -> ("command"=w9004:string, "command data"=w9003:variant)
          n4161 = call "App enquece.vi"("command data"=w9003, "command"=w9004, "queue in"=w9006) -> ("error out"=w9002:errorcluster)  [unwired: 7 in, 1 out]
        }
        n4162 = Merge Errors(w8968, w8967) -> (w8966:errorcluster)
      }
      frame "Test DRV 59A" {
        w9010 = T11 {"command"="", "command data"=variant} ("element")
        w9011 = 59 ("DUT index(0-59)")
        w9042 = T11 {"command"="", "command data"=variant} ("element")
        n4163 = disable-structure shown="LOGGING==TRUE" {
          disable-tunnel: w9021 -> [w9057 _]
          frame condition #0 (active) {
            n4164 = Empty String/Path?(string/path=w9057) -> (empty?=w9060:bool)
            n4165 = Select(t="Quece timeout", s=w9060, f=w9057) -> (s? t:f=w9056:string)
            n4166 = call "string log (SubVI).vi"("Enum"=enum16{"Init", "Log", "Read"}."Log", "state Name"=w9056) -> ()  [unwired: 8 in, 2 out]
          }
          frame condition #1 {
          }
        }
        n4167 = Flush Queue(queue=w9022) -> (queue out=w9023:refnum<queue>)  [unwired: 1 in, 2 out]
        n4168 = Decrement(x=w9011) -> (x-1=w9015:i32)
        n4169 = Index Array(array=w9012, index=w9015) -> (element=w9013:refnum<vi>)
        n4170 = property class="ColBox"(reference=w9013, "Value"=u32 10000536 ("DRV 1")) -> ()  [unwired: 1 in, 2 out]
        n4171 = To Variant(anything=T5."mux10_1_channel10" ("mux10_1(x6)_encode")) -> (Variant=w9048:variant)
        n4172 = To Variant(anything=T4."mux6_1_channel5_3" ("mux6_1(3wires)_encode")) -> (Variant=w9046:variant)
        n4173 = To Variant(anything=T6."demux1_10_channel10" ("demux1_10(x6)_encode")) -> (Variant=w9043:variant)
        n4174 = To Variant(anything=bool[] [FALSE, FALSE, FALSE, FALSE, TRUE, FALSE]) -> (Variant=w9039:variant)
        n4175 = Bundle By Name(cluster=w9042, "command"="MEAS.mux10-1", "command data"=w9048) -> (w9037:T11)
        n4176 = Bundle By Name(cluster=w9042, "command"="MEAS.mux6_1", "command data"=w9046) -> (w9036:T11)
        n4177 = Bundle By Name(cluster=w9042, "command"="MEAS.demux1-10", "command data"=w9043) -> (w9035:T11)
        n4178 = Bundle By Name(cluster=w9042, "command"="MEAS.eMIC", "command data"=w9039) -> (w9034:T11)
        n4179 = Bundle By Name(cluster=w9042, "command"="MEAS.AllRelaysOFF") -> (w9038:T11)
        n4180 = Build Array(w9038, w9037, w9036, w9035, w9034) -> (w9030:T11[])
        n4181 = Bundle By Name(cluster=w9010, "command"="MEAS.requestAC", "command data"=w9011) -> (w9031:T11)
        n4182 = Bundle By Name(cluster=w9010, "command"="Apps.WaitForEvent", "command data"=w9011) -> (w9017:T11)
        n4183 = Bundle By Name(cluster=w9010, "command"="MEAS.DMM dual read") -> (w9009:T11)
        n4184 = Bundle By Name(cluster=w9010, "command"="WaitFor") -> (w9008:T11)
        n4185 = Bundle By Name(cluster=w9010, "command"="Apps.UI Update 1") -> (w9018:T11)
        n4186 = Build Array(w9009, w9008, w9031, w9017, w9018) -> (w9029:T11[])
        n4187 = Build Array (concatenate)(w9030, w9029) -> (w9028:T11[])
        n4188 = for {
          tunnel: w9028 -> [w9064] mode=indexing
          tunnel: w9023 -> [w9065]
          tunnel: [w9061] -> w9026 mode=indexing
          n4189 = Unbundle By Name(w9064) -> ("command"=w9063:string, "command data"=w9062:variant)
          n4190 = call "App enquece.vi"("command data"=w9062, "command"=w9063, "queue in"=w9065) -> ("error out"=w9061:errorcluster)  [unwired: 7 in, 1 out]
        }
        n4191 = Merge Errors(w9027, w9026) -> (w9025:errorcluster)
      }
      frame "Test DRV 60A" {
        w9067 = T11 {"command"="", "command data"=variant} ("element")
        w9070 = 60 ("DUT index(0-59)")
        w9101 = T11 {"command"="", "command data"=variant} ("element")
        n4192 = disable-structure shown="LOGGING==TRUE" {
          disable-tunnel: w9080 -> [w9116 _]
          frame condition #0 (active) {
            n4193 = Empty String/Path?(string/path=w9116) -> (empty?=w9119:bool)
            n4194 = Select(t="Quece timeout", s=w9119, f=w9116) -> (s? t:f=w9115:string)
            n4195 = call "string log (SubVI).vi"("Enum"=enum16{"Init", "Log", "Read"}."Log", "state Name"=w9115) -> ()  [unwired: 8 in, 2 out]
          }
          frame condition #1 {
          }
        }
        n4196 = Flush Queue(queue=w9081) -> (queue out=w9082:refnum<queue>)  [unwired: 1 in, 2 out]
        n4197 = Decrement(x=w9070) -> (x-1=w9074:i32)
        n4198 = Index Array(array=w9071, index=w9074) -> (element=w9072:refnum<vi>)
        n4199 = property class="ColBox"(reference=w9072, "Value"=u32 10000536 ("DRV 1")) -> ()  [unwired: 1 in, 2 out]
        n4200 = To Variant(anything=bool[] [FALSE, FALSE, FALSE, FALSE, FALSE, TRUE]) -> (Variant=w9098:variant)
        n4201 = To Variant(anything=T6."demux1_10_channel10" ("demux1_10(x6)_encode")) -> (Variant=w9102:variant)
        n4202 = To Variant(anything=T4."mux6_1_channel6_3" ("mux6_1(3wires)_encode")) -> (Variant=w9105:variant)
        n4203 = To Variant(anything=T5."mux10_1_channel10" ("mux10_1(x6)_encode")) -> (Variant=w9107:variant)
        n4204 = Bundle By Name(cluster=w9101, "command"="MEAS.mux10-1", "command data"=w9107) -> (w9096:T11)
        n4205 = Bundle By Name(cluster=w9101, "command"="MEAS.mux6_1", "command data"=w9105) -> (w9095:T11)
        n4206 = Bundle By Name(cluster=w9101, "command"="MEAS.demux1-10", "command data"=w9102) -> (w9094:T11)
        n4207 = Bundle By Name(cluster=w9101, "command"="MEAS.eMIC", "command data"=w9098) -> (w9093:T11)
        n4208 = Bundle By Name(cluster=w9101, "command"="MEAS.AllRelaysOFF") -> (w9097:T11)
        n4209 = Build Array(w9097, w9096, w9095, w9094, w9093) -> (w9089:T11[])
        n4210 = Bundle By Name(cluster=w9067, "command"="MEAS.requestAC", "command data"=w9070) -> (w9090:T11)
        n4211 = Bundle By Name(cluster=w9067, "command"="Apps.WaitForEvent", "command data"=w9070) -> (w9076:T11)
        n4212 = Bundle By Name(cluster=w9067, "command"="MEAS.DMM dual read") -> (w9068:T11)
        n4213 = Bundle By Name(cluster=w9067, "command"="WaitFor") -> (w9066:T11)
        n4214 = Bundle By Name(cluster=w9067, "command"="Apps.UI Update 1") -> (w9077:T11)
        n4215 = Build Array(w9068, w9066, w9090, w9076, w9077) -> (w9088:T11[])
        n4216 = Build Array (concatenate)(w9089, w9088) -> (w9087:T11[])
        n4217 = for {
          tunnel: w9087 -> [w9123] mode=indexing
          tunnel: w9082 -> [w9124]
          tunnel: [w9120] -> w9085 mode=indexing
          n4218 = Unbundle By Name(w9123) -> ("command"=w9122:string, "command data"=w9121:variant)
          n4219 = call "App enquece.vi"("command data"=w9121, "command"=w9122, "queue in"=w9124) -> ("error out"=w9120:errorcluster)  [unwired: 7 in, 1 out]
        }
        n4220 = Merge Errors(w9086, w9085) -> (w9084:errorcluster)
      }
    }
